vi "Untitled 2.vi"   [LabVIEW 2018]
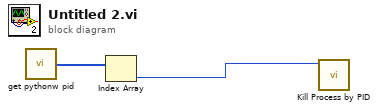
[diagram p0: block diagram]
diagram:
  n1 = call "get pythonw pid.vi"() -> ("PIDs"=w2:i32[])  [unwired: 4 in, 1 out]
  n2 = Index Array(array=w2) -> (element=w1:i32)  [unwired: 1 in]
  n3 = call "Kill Process by PID.vi"("PID"=w1) -> ()  [unwired: 10 in, 1 out]
